vi "Discrete Limited Integrator (DBL).vi"(0 "input point":dbl format="%.2f", 1 "initial condition":dbl format="%.2f", 2 "upper bound":dbl format="%.2f", 3 "lower bound":dbl format="%.2f", 4 "initialize":bool) -> (5 "output point":dbl format="%.2f")   [LabVIEW 2020, in "NI_AdvCtrl_discrete linear.lvlib"]
doc: "LabVIEW no longer supports this VI. You can obtain similar functionality by installing the LabVIEW Simulation Module.\n\nIntegrates a discrete input signal. The result of the discrete integration is limited by the lower and upper bound."
uses:
  <vilib>/addons/control/advanced/NI_AdvCtrl_discrete linear.lvlib
  <vilib>/addons/control/advanced/NI_AdvCtrl_continuous linear.lvlib
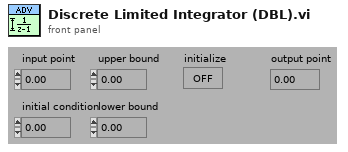
[diagram p1: front panel]
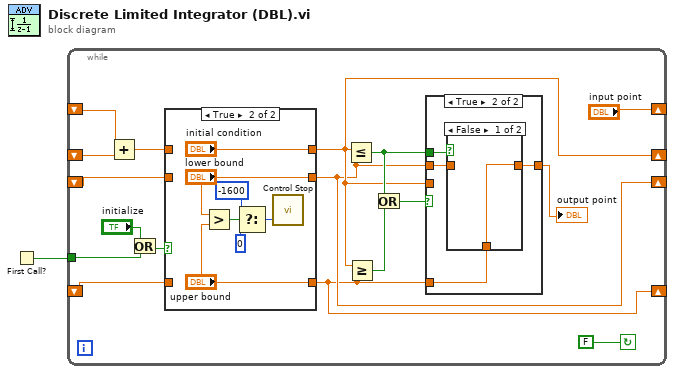
[diagram p0: block diagram]
diagram:
  n1 = First Call?() -> (First Call?: T/F=w1:bool)
  n2 = while {
    shift-left: _ -> [w3]
    shift-right: [w4] -> _
    shift-left: _ -> [w2]
    shift-right: [w5] -> _
    shift-left: _ -> [w15]
    shift-right: ["input point"] -> _
    tunnel: w1 -> [w16]
    shift-left: _ -> [w12]
    shift-right: [w7] -> _
    stop <- FALSE continue-if-true
    n3 = Add(x=w15, y=w12) -> (x+y=w6:dbl)
    n4 = Or(x="initialize", y=w16) -> (x .or. y?=w8:bool)
    n5 = case shown="True" w8 {
      tunnel: [w21 "initial condition"] -> w7
      tunnel: w6 -> [w21 _]
      tunnel: [w19 "lower bound"] -> w5
      tunnel: [w20 "upper bound"] -> w4
      tunnel: w3 -> [w20 _]
      tunnel: w2 -> [w19 _]
      frame False {
      }
      frame True {
        n6 = Greater?(x="lower bound", y="upper bound") -> (0:w25:bool)
        n7 = Select(t=-1600, s=w25, f=0) -> (s? t:f=w22:i32)
        n8 = call <vilib>:"Control Stop.vi"("error"=w22) -> ()  [unwired: 2 out]
      }
    }
    n9 = Less Or Equal?(x=w7, y=w5) -> (x <= y?=w10:bool)
    n10 = Greater Or Equal?(x=w7, y=w4) -> (x >= y?=w9:bool)
    n11 = Or(x=w10, y=w9) -> (x .or. y?=w11:bool)
    n12 = case shown="True" w11 {
      tunnel: [w29 w31] -> w13
      tunnel: w7 -> [w29 _]
      tunnel: w10 -> [_ w33]
      tunnel: w5 -> [_ w32]
      tunnel: w4 -> [_ w30]
      frame False {
      }
      frame True {
        n13 = case shown="False" w33 {
          tunnel: w32 -> [_ w35]
          tunnel: [w34 w35] -> w31
          tunnel: w30 -> [w34 _]
          frame False {
          }
          frame True {
          }
        }
      }
    }
    "output point" <- w13
  }
